vi "Set Range.vi"(2 "Range #":string, 3 "VISA Refnum in":refnum<visa-resource-name>) -> (1 "VISA Refnum out":refnum<visa-resource-name>)   [LabVIEW 2015]
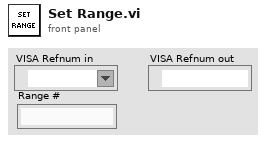
[diagram p1: front panel]
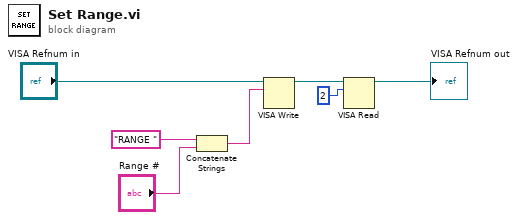
[diagram p0: block diagram]
diagram:
  n1 = Concatenate Strings("RANGE ", "Range #") -> (w1:string)
  n2 = VISA Write(VISA resource name="VISA Refnum in", write buffer=w1) -> (VISA resource name out=w6:refnum<visa-resource-name>)  [unwired: 1 in, 2 out]
  n3 = VISA Read(VISA resource name=w6, byte count=u32 2) -> (VISA resource name out=→"VISA Refnum out":refnum<visa-resource-name>)  [unwired: 1 in, 3 out]
